vi "Switch Configuration - Save Switch Configuration.vi"(8 "error in (no error)":errorcluster, 11 "Switch Config UI Data In":T1 {"Switch Config Page Item Ref" format="%.0x"}) -> (0 "error out":errorcluster, 3 "Switch Config UI Data Out":T1 {"Switch Config Page Item Ref" format="%.0x"})   [LabVIEW 2015, in "DMM-SWITCH-ScanList System Explorer.lvlib"]
doc: "This VI is called when user presses Save button. All values and relevant controls and indicators properties are saved into their corresponding Channel Properties. If user moves to another configuration page, this values will be updated in controls and indicators when selecting again Switch Configuration Page. \nChannels will also be updated. Current channels will be deleted and new channels will be created based on current Switch Configuration."
uses:
  DMM-SWITCH-ScanList System Explorer.lvlib
  Configuration Controls/Switch Config VI UI Data.ctl
  Configuration Controls/Switch Config VI UI Ctrl Values.ctl
  Configuration Controls/Switch Config VI UI Ctrl References.ctl
  <instrlib>/niSwitch/niSwitch.LLB/niSwitch Topologies.ctl
  <vilib>/NI Veristand/Custom Device API/Custom Device Item Ref.ctl
  Shared/Constants.vi
  <vilib>/NI Veristand/Custom Device API/Set Item Property (String).vi
  <vilib>/NI Veristand/Custom Device API/Set Item Property (Boolean).vi
  <vilib>/NI Veristand/Custom Device API/Set Item Property (String Array).vi
  <vilib>/NI Veristand/Custom Device API/Custom Device API.lvlib
  Shared/DMM-SWITCH-ScanList Shared.lvlib
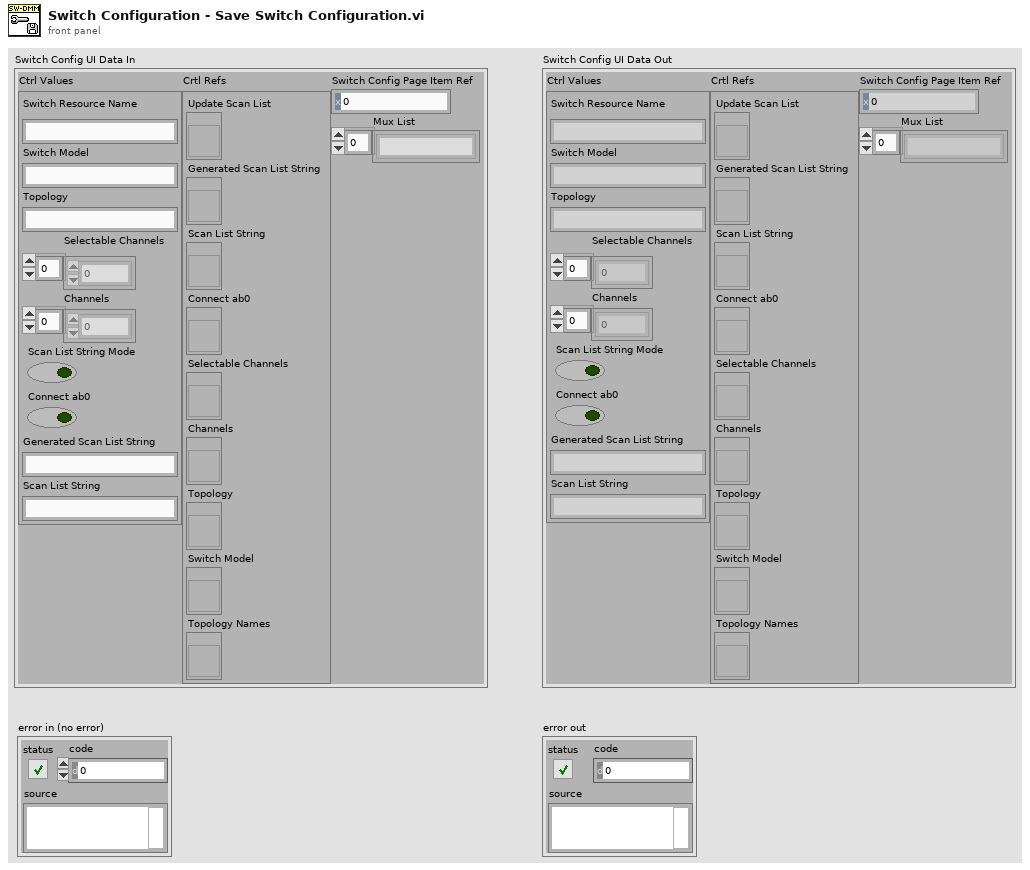
[diagram p1: front panel]
types:
  T1 = typedef "DMM-SWITCH-ScanList System Explorer.lvlib/Switch Config VI UI Data.ctl" = cluster{"Ctrl Values":T2, "Crtl Refs":T3, "Switch Config Page Item Ref":T4, "Mux List":string[]}
  T2 = typedef "DMM-SWITCH-ScanList System Explorer.lvlib/Switch Config VI UI Ctrl Values.ctl" = cluster{"Switch Resource Name":string, "Switch Model":string, "Topology":string, "Selectable Channels":i32[], "Channels":i32[], "Scan List String Mode":bool, "Connect ab0":bool, "Generated Scan List String":string, "Scan List String":string}
  T3 = typedef "DMM-SWITCH-ScanList System Explorer.lvlib/Switch Config VI UI Ctrl References.ctl" = cluster{"Update Scan List":refnum<vi>, "Generated Scan List String":refnum<vi>, "Scan List String":refnum<vi>, "Connect ab0":refnum<vi>, "Selectable Channels":refnum<vi>, "Channels":refnum<vi>, "Topology":refnum<vi>, "Switch Model":refnum<vi>, "Topology Names":refnum<vi>}
  T4 = typedef "Custom Device API.lvlib/Custom Device Item Ref.ctl" = u64
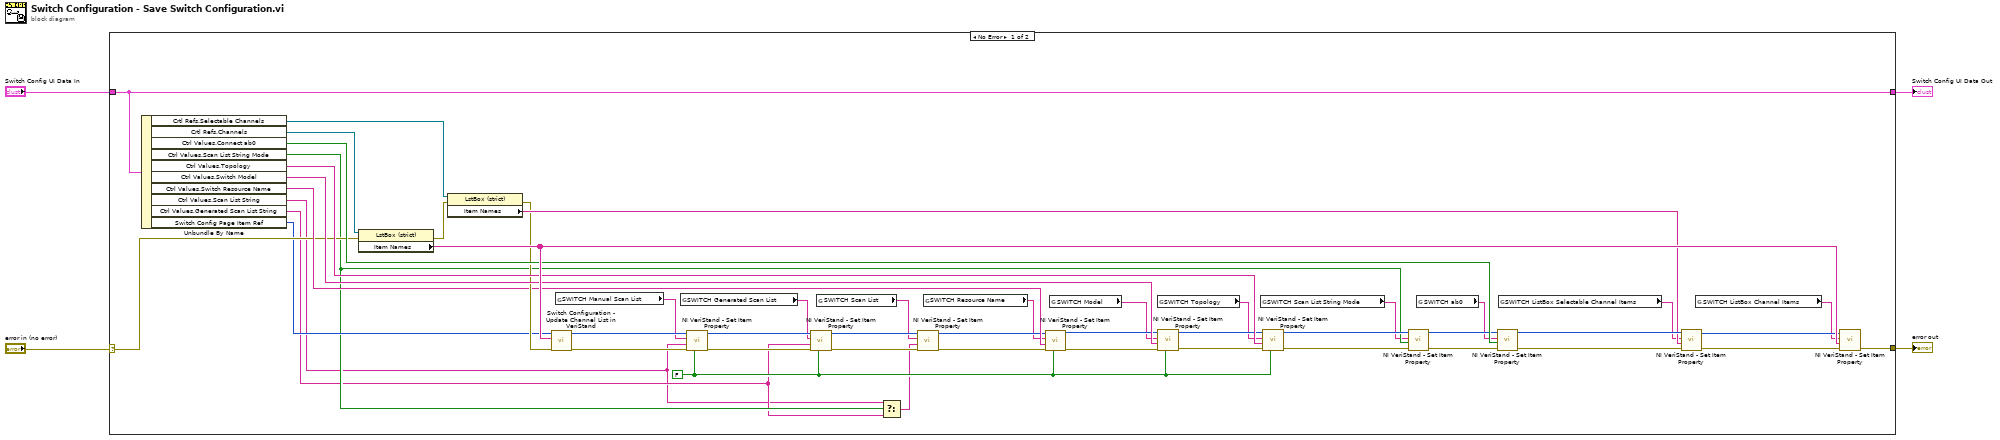
[diagram p0: block diagram]
diagram:
  n1 = case shown="No Error" "error in (no error)" {
    selector: "error in (no error)" -> [w28 w55]
    tunnel: "Switch Config UI Data In" -> [w15 w54]
    tunnel: [w32 w55] -> w3
    tunnel: [w15 w54] -> w1
    frame No Error {
      w24 = FALSE ("Binary String (T)")
      n2 = Unbundle By Name(w15) -> ("Crtl Refs.Selectable Channels"=w48:refnum<vi>, "Crtl Refs.Channels"=w47:refnum<vi>, "Ctrl Values.Connect ab0"=w49:bool, "Ctrl Values.Scan List String Mode"=w19:bool, "Ctrl Values.Topology"=w50:string, "Ctrl Values.Switch Model"=w51:string, "Ctrl Values.Switch Resource Name"=w29:string, "Ctrl Values.Scan List String"=w17:string, "Ctrl Values.Generated Scan List String"=w18:string, "Switch Config Page Item Ref"=w27:T4)
      n3 = property class="LstBox (strict)"(reference=w47, error in=w28) -> (error out=w33:errorcluster, "Item Names"=w52:string[])  [unwired: 1 out]
      n4 = property class="LstBox (strict)"(reference=w48, error in=w33) -> (error out=w34:errorcluster, "Item Names"=w35:string[])  [unwired: 1 out]
      n5 = call "Switch Configuration - Update Channel List in VeriStand.vi"("error in (no error)"=w34, "Item Names"=w52, "Item Ref In"=w27) -> ("error out"=w40:errorcluster, "Item Ref Out"=w53:T4)  [unwired: 7 in]
      n6 = global read "Constants.vi" "SWITCH Manual Scan List"() -> (w14:string)
      n7 = global read "Constants.vi" "SWITCH Generated Scan List"() -> (w13:string)
      n8 = call-poly <vilib>:"NI VeriStand - Set Item Property.vi"("Binary String (T)"=w24, "error in (no error)"=w40, "Value"=w17, "Property Name"=w14, "Item Ref in"=w53) -> ("error out"=w25:errorcluster, "Item Ref out"=w26:T4)  [unwired: 4 in, 1 out]
      n9 = call-poly <vilib>:"NI VeriStand - Set Item Property.vi"("Binary String (T)"=w24, "error in (no error)"=w25, "Value"=w18, "Property Name"=w13, "Item Ref in"=w26) -> ("error out"=w22:errorcluster, "Item Ref out"=w23:T4)  [unwired: 4 in, 1 out]
      n10 = global read "Constants.vi" "SWITCH Scan List"() -> (w12:string)
      n11 = Select(t=w17, s=w19, f=w18) -> (s? t:f=w16:string)
      n12 = call-poly <vilib>:"NI VeriStand - Set Item Property.vi"("error in (no error)"=w22, "Value"=w16, "Property Name"=w12, "Item Ref in"=w23) -> ("error out"=w21:errorcluster, "Item Ref out"=w20:T4)  [unwired: 5 in, 1 out]
      n13 = global read "Constants.vi" "SWITCH Resource Name"() -> (w11:string)
      n14 = call-poly <vilib>:"NI VeriStand - Set Item Property.vi"("Binary String (T)"=w24, "error in (no error)"=w21, "Value"=w29, "Property Name"=w11, "Item Ref in"=w20) -> ("error out"=w36:errorcluster, "Item Ref out"=w38:T4)  [unwired: 4 in, 1 out]
      n15 = global read "Constants.vi" "SWITCH Model"() -> (w10:string)
      n16 = global read "Constants.vi" "SWITCH Topology"() -> (w9:string)
      n17 = call-poly <vilib>:"NI VeriStand - Set Item Property.vi"("Binary String (T)"=w24, "error in (no error)"=w36, "Value"=w51, "Property Name"=w10, "Item Ref in"=w38) -> ("error out"=w37:errorcluster, "Item Ref out"=w39:T4)  [unwired: 4 in, 1 out]
      n18 = global read "Constants.vi" "SWITCH Scan List String Mode"() -> (w8:string)
      n19 = call-poly <vilib>:"NI VeriStand - Set Item Property.vi"("Binary String (T)"=w24, "error in (no error)"=w37, "Value"=w50, "Property Name"=w9, "Item Ref in"=w39) -> ("error out"=w44:errorcluster, "Item Ref out"=w43:T4)  [unwired: 4 in, 1 out]
      n20 = call-poly <vilib>:"NI VeriStand - Set Item Property.vi"("error in (no error)"=w44, "Value"=w19, "Property Name"=w8, "Item Ref in"=w43) -> ("error out"=w46:errorcluster, "Item Ref out"=w41:T4)  [unwired: 5 in, 1 out]
      n21 = global read "Constants.vi" "SWITCH ab0"() -> (w7:string)
      n22 = call-poly <vilib>:"NI VeriStand - Set Item Property.vi"("error in (no error)"=w46, "Value"=w49, "Property Name"=w7, "Item Ref in"=w41) -> ("error out"=w45:errorcluster, "Item Ref out"=w42:T4)  [unwired: 5 in, 1 out]
      n23 = global read "Constants.vi" "SWITCH ListBox Selectable Channel Items"() -> (w6:string)
      n24 = call-poly <vilib>:"NI VeriStand - Set Item Property.vi"("error in (no error)"=w45, "Value"=w35, "Property Name"=w6, "Item Ref in"=w42) -> ("error out"=w30:errorcluster, "Item Ref out"=w31:T4)  [unwired: 5 in, 1 out]
      n25 = global read "Constants.vi" "SWITCH ListBox Channel Items"() -> (w5:string)
      n26 = call-poly <vilib>:"NI VeriStand - Set Item Property.vi"("error in (no error)"=w30, "Value"=w52, "Property Name"=w5, "Item Ref in"=w31) -> ("error out"=w32:errorcluster)  [unwired: 5 in, 2 out]
    }
    frame Error {
    }
  }
  "error out" <- w3
  "Switch Config UI Data Out" <- w1
